vi "Get Attribute Name and Parent ID.vi"(8 "error in (no error)":errorcluster, 10 "Tag":string, 11 "Test Executive Ref":refnum<data-value>) -> (0 "error out":errorcluster, 1 "Attribute Name":string, 2 "Parent ID":string, 3 "Test Executive Ref out":refnum<data-value>)   [LabVIEW 2020, in "Test Executive.lvlib" / "TestExecutive Ref.lvclass"]
uses:
  <vilib>/gpm_packages/@cs/test-executive/Source/Test Executive/TestExecutive Ref/TestExecutive Ref.lvclass
  <vilib>/gpm_packages/@cs/test-executive/Source/Test Executive/ITestExecutive/ITest Executive.lvclass
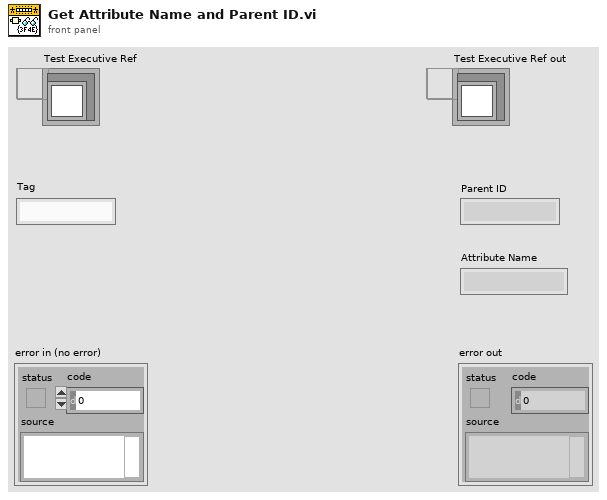
[diagram p1: front panel]
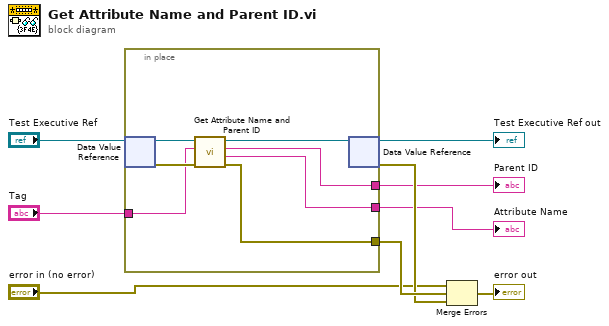
[diagram p0: block diagram]
diagram:
  n1 = in-place {
    in-place-border: [w13] -> w9
    in-place-border: [w12] -> w2
    in-place-border: [w11] -> w1
    in-place-border: "Tag" -> [w10]
    n2 = in-place-dvr #1("Test Executive Ref") -> (w16:refnum<class "ITest Executive.lvclass">, w14:errorcluster)
    n3 = call-dynamic "Get Attribute Name and Parent ID.vi"("error in (no error)"=w14, "Tag"=w10, "ITest Executive in"=w16) -> ("error out"=w13:errorcluster, "Attribute Name"=w11:string, "Parent ID"=w12:string, "ITest Executive out"=w15:refnum<class "ITest Executive.lvclass">)  [unwired: 5 in]
    n4 = in-place-dvr #1(w15) -> (→"Test Executive Ref out":refnum<data-value>, w8:errorcluster)
  }
  "Parent ID" <- w2
  "Attribute Name" <- w1
  n5 = Merge Errors("error in (no error)", w9, w8) -> (→"error out":errorcluster)
